vi "Set Data on Point.vi"(0 "eye scan point iterator":refnum<class "niHighSpeedSerial Eye Scan Point Iterator v1 Host.lvclass">, 5 "bit error ratio":dbl, 7 "sample count":u64, 9 "error count":u64, 11 "error in":errorcluster) -> (4 "eye scan point iterator out":refnum<class "niHighSpeedSerial Eye Scan Point Iterator v1 Host.lvclass">, 15 "error out":errorcluster)   [LabVIEW 2014, in "niHighSpeedSerial Eye Scan Point Iterator v1 Host.lvclass"]
doc: "Sets the specified data on the active point.\n\n<B>Input Parameters</B>\n\n<B>eye scan point iterator</B> is the incoming wire for the Eye Scan Point Iterator class object\n\n<B>bit error rate</B> is the calculated statistical bit error rate based on the number of error counts and sample counts received.\n\n<B>sample count</B> is the number of samples that have been measured on this point.\n\n<B>error count</B> is the number of errors that have been measured on this point.\n\n<B>error in</B> describes error conditions that occur before this node runs. This input provides standard 'error in' functionality.\n\n<B>Output Parameters</B>\n\n<B>eye scan point iterator out</B> is the outgoing wire for the Eye Scan Point Iterator class object\n\n<B>error out</B> contains error information. This output provides standard 'error out' functionality."
uses:
  <instrlib>/niHighSpeedSerial/Eye Scan/v1/Host/Impl/Eye Scan Point Iterator/niHighSpeedSerial Eye Scan Point Iterator v1 Host.lvclass
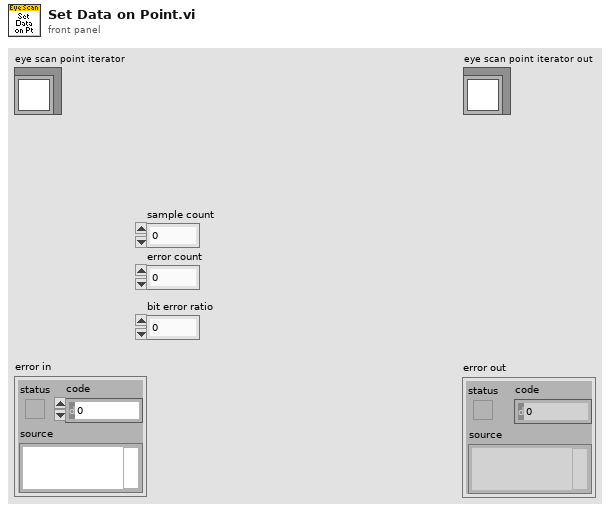
[diagram p1: front panel]
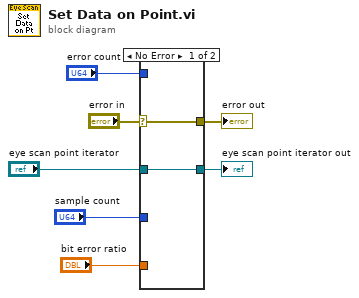
[diagram p0: block diagram]
diagram:
  n1 = case shown="No Error" "error in" {
    selector: "error in" -> [w8 w11]
    tunnel: [w8 w11] -> w6
    tunnel: [w9 w10] -> w4
    tunnel: "eye scan point iterator" -> [w9 w10]
    tunnel: "error count" -> [_ _]
    tunnel: "sample count" -> [_ _]
    tunnel: "bit error ratio" -> [_ _]
    frame No Error {
    }
    frame Error {
    }
  }
  "error out" <- w6
  "eye scan point iterator out" <- w4
